vi "Echo.vi"(8 "error in (no error)":errorcluster, 10 "Audio Data In":dbl[][](array[numeric]), 11 "Effect in":refnum<class "Effect.lvclass">) -> (0 "error out":errorcluster, 2 "Audio Data Out":dbl[][](array[numeric]), 3 "Effect out":refnum<class "Effect.lvclass">)   [LabVIEW 2018, in "Effect.lvclass"]
uses:
  Effect.lvclass
  Effect.lvclass/Effect.ctl
  Libraries/Globals/Constants.vi
  Libraries/Globals/Globals.lvlib
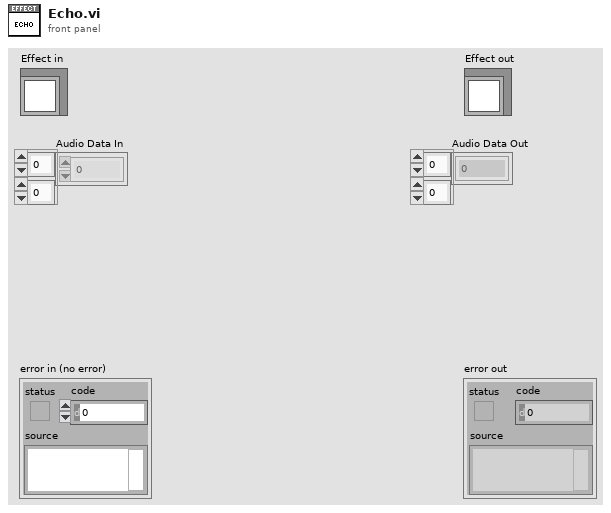
[diagram p1: front panel]
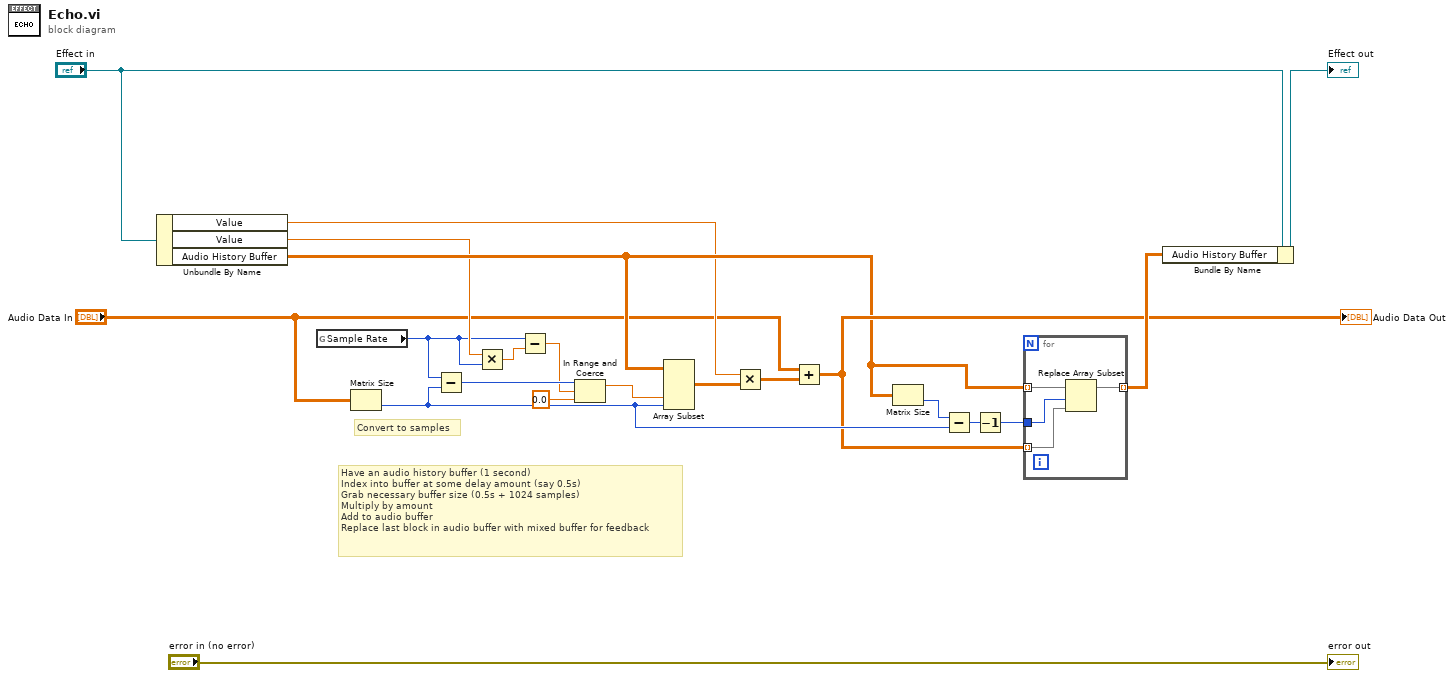
[diagram p0: block diagram]
diagram:
  # "Convert to samples"
  # "Have an audio history buffer (1 second)\nIndex into buffer at some delay amount (say 0.5s)\nGrab necessary buffer size (0.5s + 1024 samples)\nMultiply by amount\nAdd to audio buffer\nReplace last block in audio buffer with mixed buffer for feedback"
  n1 = Unbundle By Name("Effect in") -> ("Value"=w4:dbl, "Value"=w5:dbl, "Audio History Buffer"=w6:dbl[][])
  n2 = global read "Constants.vi" "Sample Rate"() -> (w1:i32)
  n3 = Matrix Size(0:"Audio Data In") -> (2:w13:i32)  [unwired: 1 out]
  n4 = Subtract(x=w1, y=w13) -> (x-y=w12:i32)
  n5 = Multiply(x=w5, y=w1) -> (x*y=w20:dbl)
  n6 = Subtract(x=w1, y=w20) -> (x-y=w11:dbl)
  n7 = In Range and Coerce(upper limit=w12, x=w11, lower limit=0.0) -> (coerced(x)=w9:dbl)  [unwired: 1 out]
  n8 = Array Subset(array=w6, index (col)=w9, length (col)=w13) -> (w19:dbl[][])  [unwired: 2 in]
  n9 = Multiply(x=w4, y=w19) -> (x*y=w18:dbl[][])
  n10 = Add(x="Audio Data In", y=w18) -> (x+y=w7:dbl[][])
  "Audio Data Out" <- w7
  n11 = Matrix Size(0:w6) -> (2:w17:i32)  [unwired: 1 out]
  n12 = Subtract(x=w17, y=w13) -> (x-y=w16:i32)
  n13 = Decrement(x=w16) -> (x-1=w14:i32)
  n14 = for {
    tunnel: w14 -> [w24]
    tunnel: w6 -> [w25] mode=indexing
    tunnel: [w23] -> w15 mode=indexing
    tunnel: w7 -> [w22] mode=indexing
    n15 = Replace Array Subset(array=w25, new element=w22, index=w24) -> (w23:dbl[])
  }
  n16 = Bundle By Name(cluster="Effect in", "Audio History Buffer"=w15) -> (→"Effect out":refnum<class "Effect.lvclass">)
  "error out" <- "error in (no error)"
